vi "dsfsdfsd_Read Array.vi"(8 "error in (no error)":errorcluster, 11 "dsfsdfsd in":refnum<class "dsfsdfsd.lvclass">) -> (0 "error out":errorcluster, 2 "Array":cluster{"Numeric":dbl, "String":string}[](array[cluster]), 3 "dsfsdfsd out":refnum<class "dsfsdfsd.lvclass">)   [LabVIEW 2013, in "dsfsdfsd.lvclass"]
uses:
  dsfsdfsd.lvclass
  dsfsdfsd.lvclass/dsfsdfsd.ctl
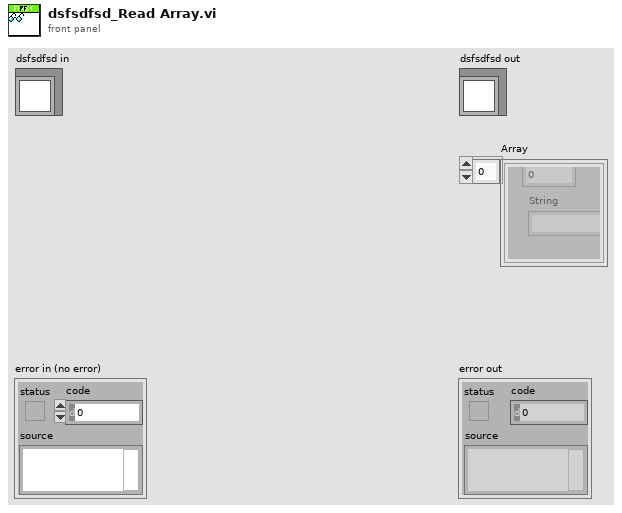
[diagram p1: front panel]
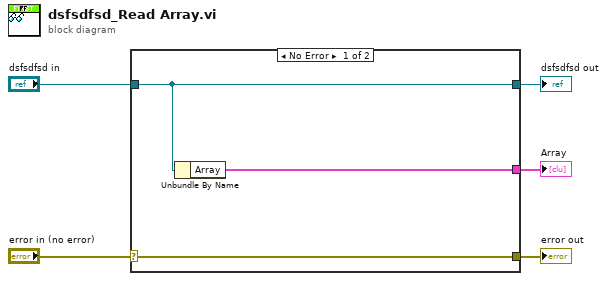
[diagram p0: block diagram]
diagram:
  n1 = case shown="No Error" "error in (no error)" {
    selector: "error in (no error)" -> [w8 w9]
    tunnel: [w8 w9] -> w4
    tunnel: [w7 w10] -> w2
    tunnel: "dsfsdfsd in" -> [w7 w10]
    tunnel: [w6 _] -> w1
    frame No Error {
      n2 = Unbundle By Name "Unbundle By Name"(w7) -> ("Array"=w6:cluster{"Numeric":dbl, "String":string}[])
    }
    frame Error {
    }
  }
  "error out" <- w4
  "dsfsdfsd out" <- w2
  "Array" <- w1
